vi "Keithley 6514 Meas Voltage Example_NEW_TIME.vi"() -> ()   [LabVIEW 2010, in "Keithley 6514 LV 2009.lvlib"]
uses:
  Keithley 6514 LV 2009.lvlib
panel:
  in  "Filename":path=path "C:/Users/Admin/Desktop/charge/test11.lvm"
  in  "stop":bool
  out "error out":T1
  out "Data Plot":sgl[](graph)
  out "Data":sgl[][](array[numeric]) format="%^.4e"
  in  "Timeout (msecs)":u32=5000
  in  "Trigger Delay":sgl min=0 max=999.9999 step=0.0001 format="%.2f"
  in  "Trigger Count":i16=10 min=1 max=2500 step=1
  in  "Autorange Lower Limit (V)":sgl=2.1 min=0 max=210 step=0.1 format="%^.2e"
  in  "Autorange Upper Limit (V)":sgl=210.0 min=0 max=210 step=0.1 format="%^.2e"
  in  "External Feedback Enabled?":bool
  in  "Driven Guard?":bool
  in  "Check For SCPI Errors?":bool=TRUE
  in  "Range Value (V)":sgl=21.0 min=0 max=210 step=0.1 format="%.2f"
  in  "Ranging Method":u16(ring) items=["autorange", "set min range", "set max range", "set range value"]
  in  "Integration Time (NPLCs)":dbl=1.0 min=0.01 max=10.0 step=0.01 format="%.2f"
  in  "Resource":refnum<visa-resource-name>
  # "Input"
  # "Output"
  # "Measurement\n(V)"
  # "Timestamp\n(secs)"
  # "Status"
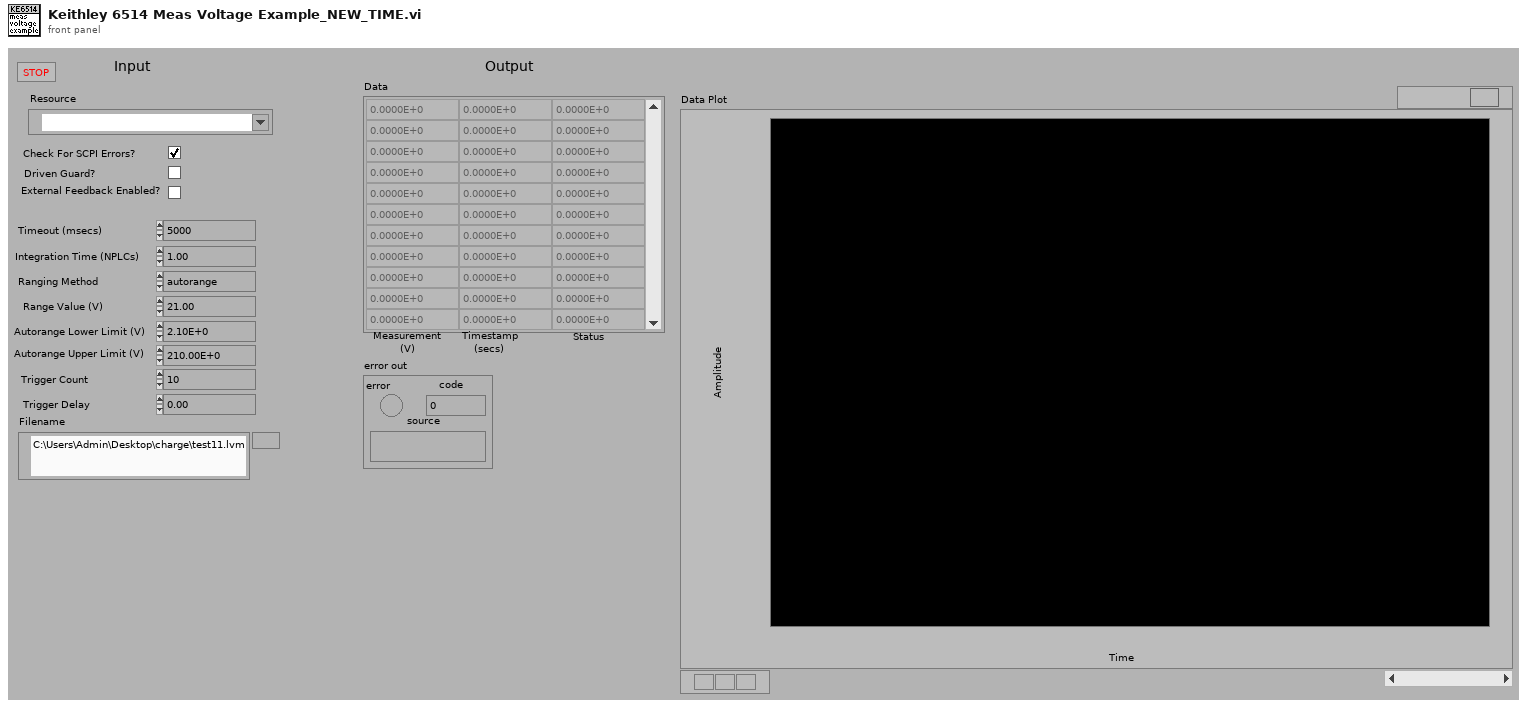
[diagram p1: front panel]
types:
  T1 = cluster{"error":bool, "code":i32, "source":string}
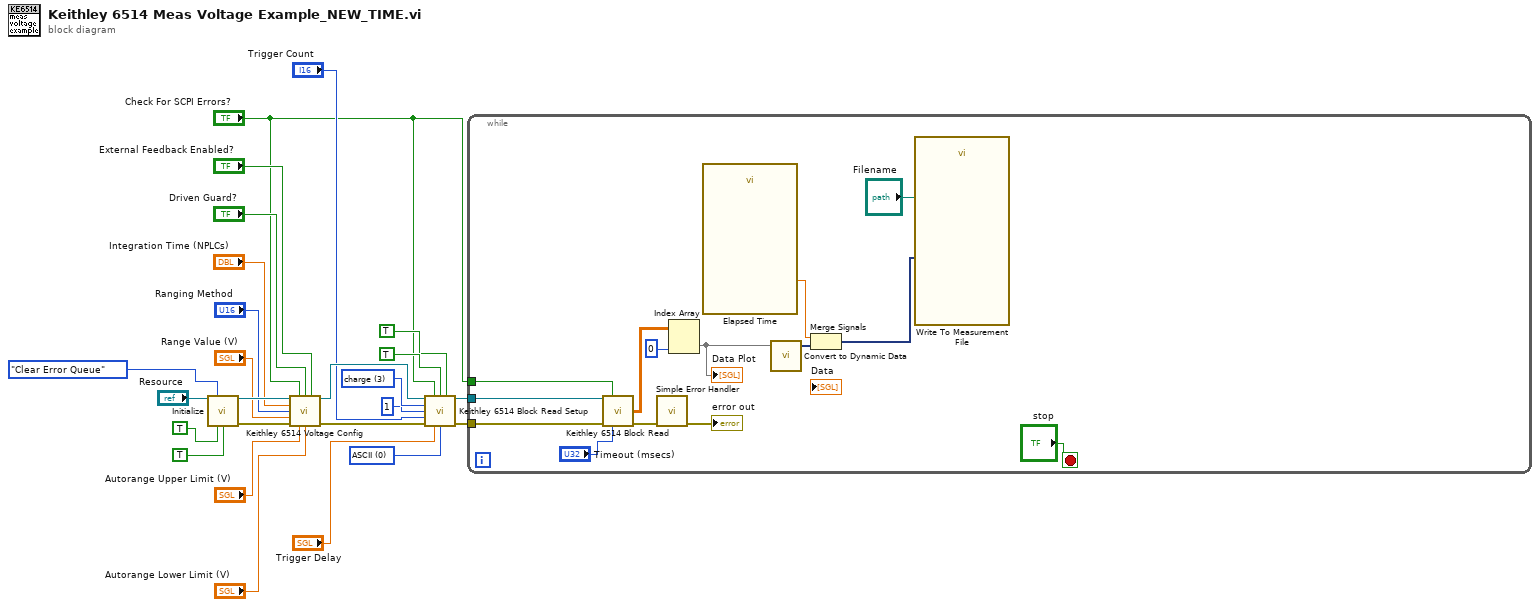
[diagram p0: block diagram]
diagram:
  w3 = u16 0 items=["ASCII", "Single Precision REAL"] ("Data Type (ASCII:0)")
  w9 = u16 3 items=["dc voltage", "resistance", "dc current", "charge"] ("function (Vdc:1)")
  n1 = call "Initialize.vi"("VISA resource name"="Resource", "Error Queue Option"=enum16{"Clear Error Queue", "Error Query"}."Clear Error Queue", "ID Query? (T)"=TRUE, "Reset? (T)"=TRUE) -> ("VISA resource name out"=w21:refnum<visa-resource-name>, "error out"=w20:errorcluster)  [unwired: 10 in]
  n2 = call "Keithley 6514 Voltage Config.vi"("Resource In"=w21, "Check For SCPI Errors? (T)"="Check For SCPI Errors?", "Driven Guard (Off:F)"="Driven Guard?", "External Feedback (Disabled:F)"="External Feedback Enabled?", "NPLC value (1.00)"="Integration Time (NPLCs)", "range (autorange:0)"="Ranging Method", "range value (V) (21)"="Range Value (V)", "error in (no error)"=w20, "Autorange Upper Limit (V) (210)"="Autorange Upper Limit (V)", "Autorange Lower Limit (V) (2.1)"="Autorange Lower Limit (V)") -> ("Resource Out (dupl)"=w12:refnum<visa-resource-name>, "error out"=w6:T1)  [unwired: 4 in]
  n3 = call "Keithley 6514 Block Read Setup.vi"("Resource In"=w12, "Check For SCPI Errors? (T)"="Check For SCPI Errors?", "Time (F)"=TRUE, "Status (F)"=TRUE, "function (Vdc:1)"=w9, "Arm Layer Count (1)"=i16 1, "Trigger Layer Count (1)"="Trigger Count", "error in (no error)"=w6, "Trigger Layer Delay (0 secs)"="Trigger Delay", "Data Type (ASCII:0)"=w3) -> ("Resource Out (dupl)"=w2:refnum<visa-resource-name>, "error out"=w1:T1)  [unwired: 4 in]
  n4 = while {
    tunnel: "Check For SCPI Errors?" -> [w39]
    tunnel: w2 -> [w37]
    tunnel: w1 -> [w36]
    stop <- "stop" stop-if-true
    n5 = call "Keithley 6514 Block Read.vi"("Resource In"=w37, "Check For SCPI Errors? (T)"=w39, "error in (no error)"=w36, "Timeout (5000 msecs)"="Timeout (msecs)") -> ("Test Data"=w31:sgl[][], "error out"=w35:T1)  [unwired: 7 in, 3 out]
    n6 = call <vilib>:"Simple Error Handler.vi"("error in (no error)"=w35) -> ("error out"=→"error out":errorcluster)  [unwired: 4 in, 4 out]
    n7 = Index Array(array=w31, index (col)=0 ("disabled index (col)")) -> (element=w27:sgl[])  [unwired: 1 in]
    "Data Plot" <- w27
    n8 = call "Elapsed Time"() -> ("Elapsed Time (s)"=w26:dbl)  [unwired: 12 in, 7 out]
    n9 = call "Convert to Dynamic Data"("Array"=w27) -> ("Dynamic Data Type"=w29:dynamicdata)  [unwired: 3 in]
    n10 = Merge Signals(w26, w29) -> (w28:dynamicdata)
    n11 = call "Write To Measurement File"("Signals"=w28, "Filename"="Filename") -> ()  [unwired: 15 in, 3 out]
  }
